vi "FetchL1Measurements.vi"(8 "error in (no error)":errorcluster, 10 "Link Direction":enum16{"Uplink", "Downlink"}(ring)=enum."Downlink", 11 "vi path":path=path "C:/g/jma-poc-clean/src/LV-RT-Host/Plug-Ins/Standard/GUI/Deploy GUI (Host).vi") -> (0 "error out":errorcluster, 1 "PHY grant":dbl, 2 "PHY CRC pass":dbl, 3 "MAC":dbl, 5 "L1 Measurements":T1)   [LabVIEW 2019]
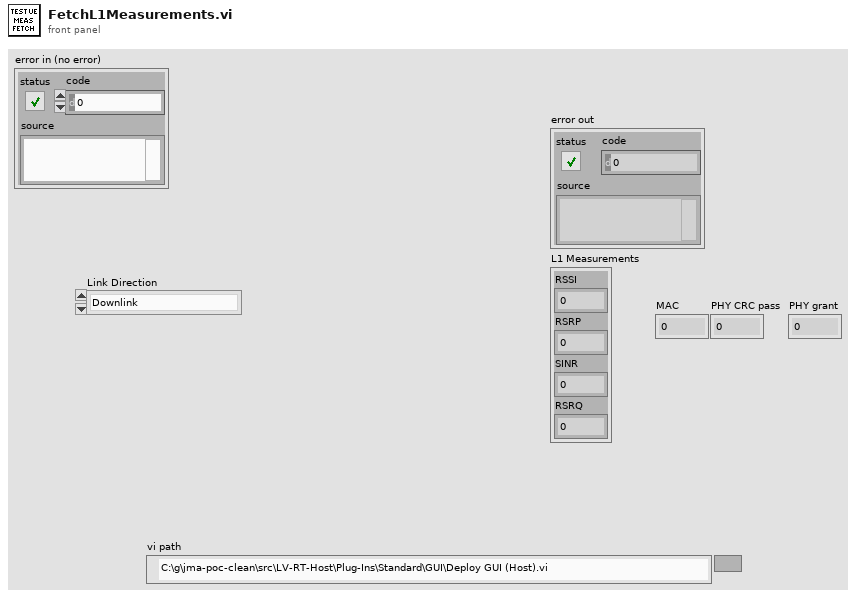
[diagram p1: front panel]
types:
  T1 = cluster{"RSSI":dbl, "RSRP":dbl, "SINR":dbl, "RSRQ":dbl}
  T2 = cluster{"MAC":dbl, "String 2":string, "color 2":u32, "PHY CRC pass":dbl, "String 3":string, "color 3":u32, "PHY grant":dbl, "String 4":string, "color 4":u32}
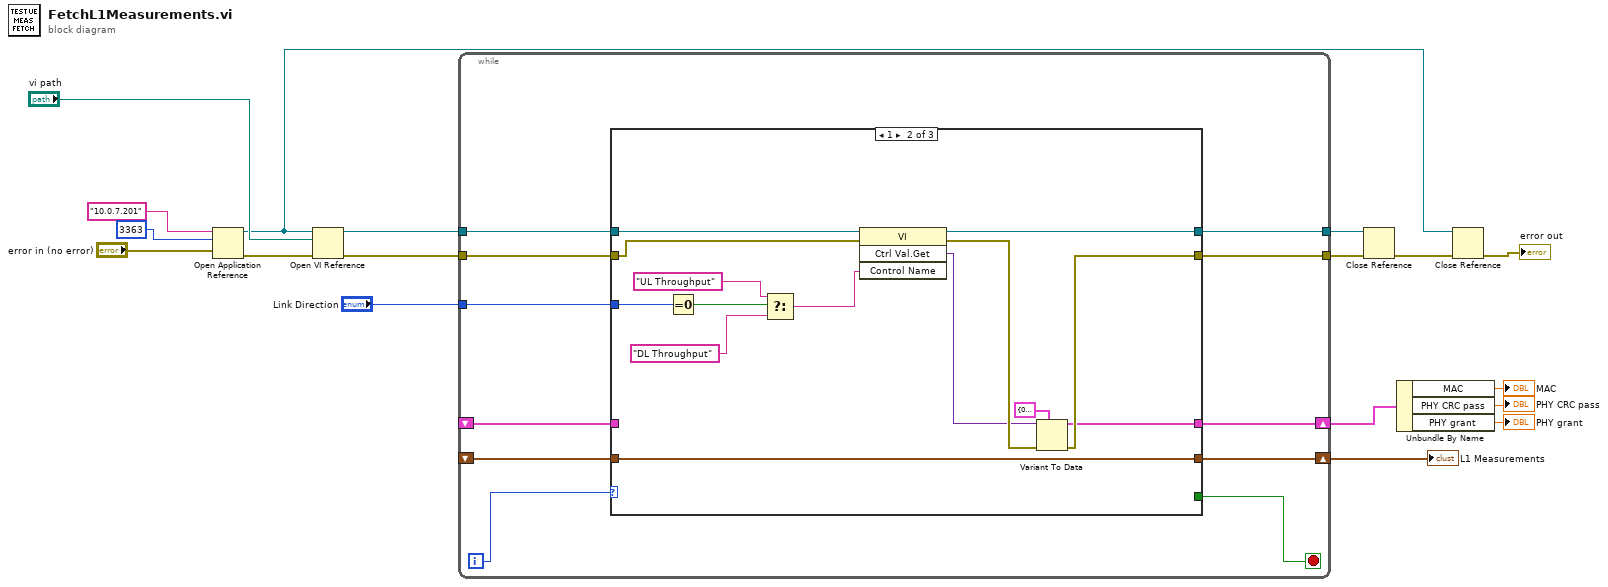
[diagram p0: block diagram]
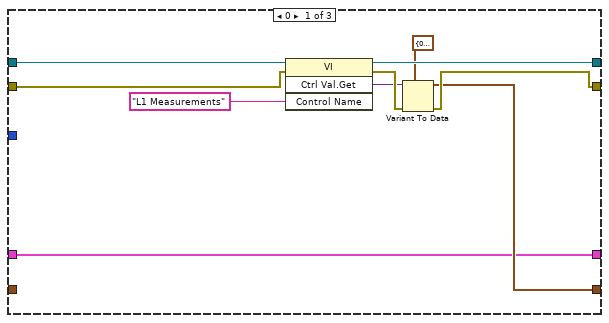
[diagram p2: hidden frame]
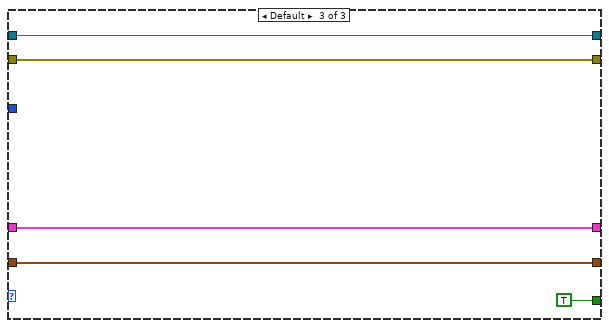
[diagram p3: hidden frame]
diagram:
  n1 = Open Application Reference(8:"error in (no error)", 10:u16 3363 ("port number or service name (3363)"), 11:"10.0.7.201" ("machine name (\"\":  open local reference)")) -> (0:w17:errorcluster, 3:w10:refnum<vi>)  [unwired: 1 in]
  n2 = Open VI Reference(application reference (local)=w10, vi path="vi path", error in (no error)=w17) -> (vi reference=w12:refnum<vi>, error out=w9:errorcluster)  [unwired: 3 in]
  n3 = while {
    tunnel: w12 -> [w28]
    tunnel: [w27] -> w11
    shift-right: [w26] -> w6
    shift-left: _ -> [w25]
    tunnel: w9 -> [w24]
    tunnel: [w23] -> w8
    tunnel: "Link Direction" -> [w22]
    shift-right: [w21] -> w5
    shift-left: _ -> [w20]
    i -> [w29]
    stop <- w19 stop-if-true
    n4 = case shown="1" w29 {
      tunnel: w28 -> [w37 w51 w55]
      tunnel: [w36 w50 w55] -> w27
      tunnel: [w32 w43 w57] -> w26
      tunnel: w25 -> [_ w43 w57]
      tunnel: w24 -> [w31 w49 w54]
      tunnel: [w38 w52 w54] -> w23
      tunnel: w22 -> [_ w48 _]
      tunnel: [w30 w40 w56] -> w21
      tunnel: w20 -> [w30 _ w56]
      tunnel: [_ _ TRUE] -> w19
      frame 0 {
        n5 = invoke class="VI" method="Ctrl Val.Get"(reference=w37, error in=w31, "Control Name"="L1 Measurements") -> (reference out=w36:refnum<vi>, error out=w39:errorcluster, "Get Control Value Variant"=w34:variant)  [unwired: 1 in, 1 out]
        n6 = Variant To Data(error in=w39, type=T1 {"RSSI"=0.0, "RSRP"=0.0, "SINR"=0.0, "RSRQ"=0.0} ("L1 Measurements"), Variant=w34) -> (data=w32:T1, error out=w38:errorcluster)
      }
      frame 1 {
        n7 = Equal To 0?(x=w48) -> (x = 0?=w47:bool)
        n8 = Select(t="UL Throughput" ("Control Name"), s=w47, f="DL Throughput" ("Control Name")) -> (s? t:f=w44:string)
        n9 = invoke class="VI" method="Ctrl Val.Get"(reference=w51, error in=w49, "Control Name"=w44) -> (reference out=w50:refnum<vi>, error out=w53:errorcluster, "Get Control Value Variant"=w42:variant)  [unwired: 1 in, 1 out]
        n10 = Variant To Data(error in=w53, type=T2 {"MAC"=0.0, "String 2"="MAC", "color 2"=16860, "PHY CRC pass"=0.0, "String 3"="PHY CRC", "color 3"=6618880, "PHY grant"=0.0, "String 4"="PHY grant", "color 4"=16711680} ("UL Throughput"), Variant=w42) -> (data=w40:T2, error out=w52:errorcluster)
      }
      frame Default {
      }
    }
  }
  "L1 Measurements" <- w6
  n11 = Close Reference(reference=w11, error in (no error)=w8) -> (error out=w14:errorcluster)
  n12 = Unbundle By Name(w5) -> ("MAC"=→"MAC":dbl, "PHY CRC pass"=→"PHY CRC pass":dbl, "PHY grant"=→"PHY grant":dbl)
  n13 = Close Reference(reference=w10, error in (no error)=w14) -> (error out=→"error out":errorcluster)
